vi "CAN_Simple_Demo.vi"() -> ()   [LabVIEW 2014]
uses:
  <vilib>/Utility/miscctls.llb/LVPointTypeDef.ctl
  Utilities/Global/DLL_Path.vi
  Utilities/Typedef/Hardware_Subtype.ctl
  TSMaster_API/CAN_CANFD_Function/Typedef/TSCAN_CAN_Configuration.ctl
  TSMaster_API/All_Control/Typedef/Hardware Type.ctl
panel:
  in  "Hardware Subtype":T1=enum."TC1016"
  in  "DLL_Path":path=path "D:/Program Files (x86)/TOSUN/TSMaster/bin/TSMaster.dll"
  out "ACANMsgBuffer":T2(array[cluster])
  out "Initialize array1":T2(array[cluster])
  out "Message&ID":string[](array[string])
  in  "Send":bool
  out "Initialize array":string[](array[string])
  out "ALLName":string[](array[string])
  out "SignalName":string[][](array[string])
  out "Message":string[](array[string])
  in  "tab control":enum32{"CANUI", "DBCUI"}(tab)
  in  "Data":T3 {"Data7" format="%x"; "Data6" format="%x"; "Data5" format="%x"; "Data4" format="%x"; "Data3" format="%x"; "Data2" format="%x"; "Data1" format="%x"; "Data0" format="%.0x"}
  in  "Length":u8
  in  "Frame type":u8(ring) items=["Data Frame", "Remote Frame"]
  in  "Frame format":u8(ring) items=["Standard Frame", "Extended Frame"]
  in  "ID 2":i32 format="%x"
  in  "Channel select":u8(ring) items=["CHN1", "CHN2", "CHN3", "CHN4", "CHN5", "CHN6", "CHN7", "CHN8", "CHN9", "CHN10", "CHN11", "CHN12", "CHN13", "CHN14", "CHN15", "CHN16", "CHN17", "CHN18", "CHN19", "CHN20", "CHN21", "CHN22", "CHN23", "CHN24", "CHN25", "CHN26", "CHN27", "CHN28", "CHN29", "CHN30", "CHN31", "CHN32"]
  in  "Data":i32(listbox)=-1
  in  "READ":i32(listbox)
  in  "Tree control":string(tree)
  in  "DBC Path":path
  in  "DBC loading channel":i32(ring) items=["CHN1", "CHN2", "CHN3", "CHN4", "CHN5", "CHN6", "CHN7", "CHN8", "CHN9", "CHN10", "CHN11", "CHN12", "CHN13", "CHN14", "CHN15", "CHN16", "CHN17", "CHN18", "CHN19", "CHN20", "CHN21", "CHN22", "CHN23", "CHN24", "CHN25", "CHN26", "CHN27", "CHN28", "CHN29", "CHN30", "CHN31", "CHN32"]
  in  "WRITE":string[][](table)
  out "ID":i32[](array[numeric]) format="%x"
  out "Connect":bool
  in  "Baud rate setting":dbl=500.0 format="%#_g k"
  in  "Application logic channel":i32(ring) items=["CHN1", "CHN2", "CHN3", "CHN4", "CHN5", "CHN6", "CHN7", "CHN8", "CHN9", "CHN10", "CHN11", "CHN12", "CHN13", "CHN14", "CHN15", "CHN16", "CHN17", "CHN18", "CHN19", "CHN20", "CHN21", "CHN22", "CHN23", "CHN24", "CHN25", "CHN26", "CHN27", "CHN28", "CHN29", "CHN30", "CHN31", "CHN32"]
  in  "Physical channel":i32(ring) items=["CHN1", "CHN2", "CHN3", "CHN4", "CHN5", "CHN6", "CHN7", "CHN8", "CHN9", "CHN10", "CHN11", "CHN12", "CHN13", "CHN14", "CHN15", "CHN16", "CHN17", "CHN18", "CHN19", "CHN20", "CHN21", "CHN22", "CHN23", "CHN24", "CHN25", "CHN26", "CHN27", "CHN28", "CHN29", "CHN30", "CHN31", "CHN32"]
  in  "Terminator":u16(ring)=1 items=["Disable", "Enable"]
  in  "Mode":u16(ring) items=["Normal", "ListenOnly"]
  in  "Number of channels used":u16(ring)=1 items=["1 Channel"=1, "2 Channels"=2, "3 Channels"=3, "4 Channels"=4, "5 Channels"=5]
  in  "Read message type":u16(ring)=1 items=["Only read received messages", "Receive&send messages"]
  in  "Hardware on/off":bool
  in  "Exit":bool
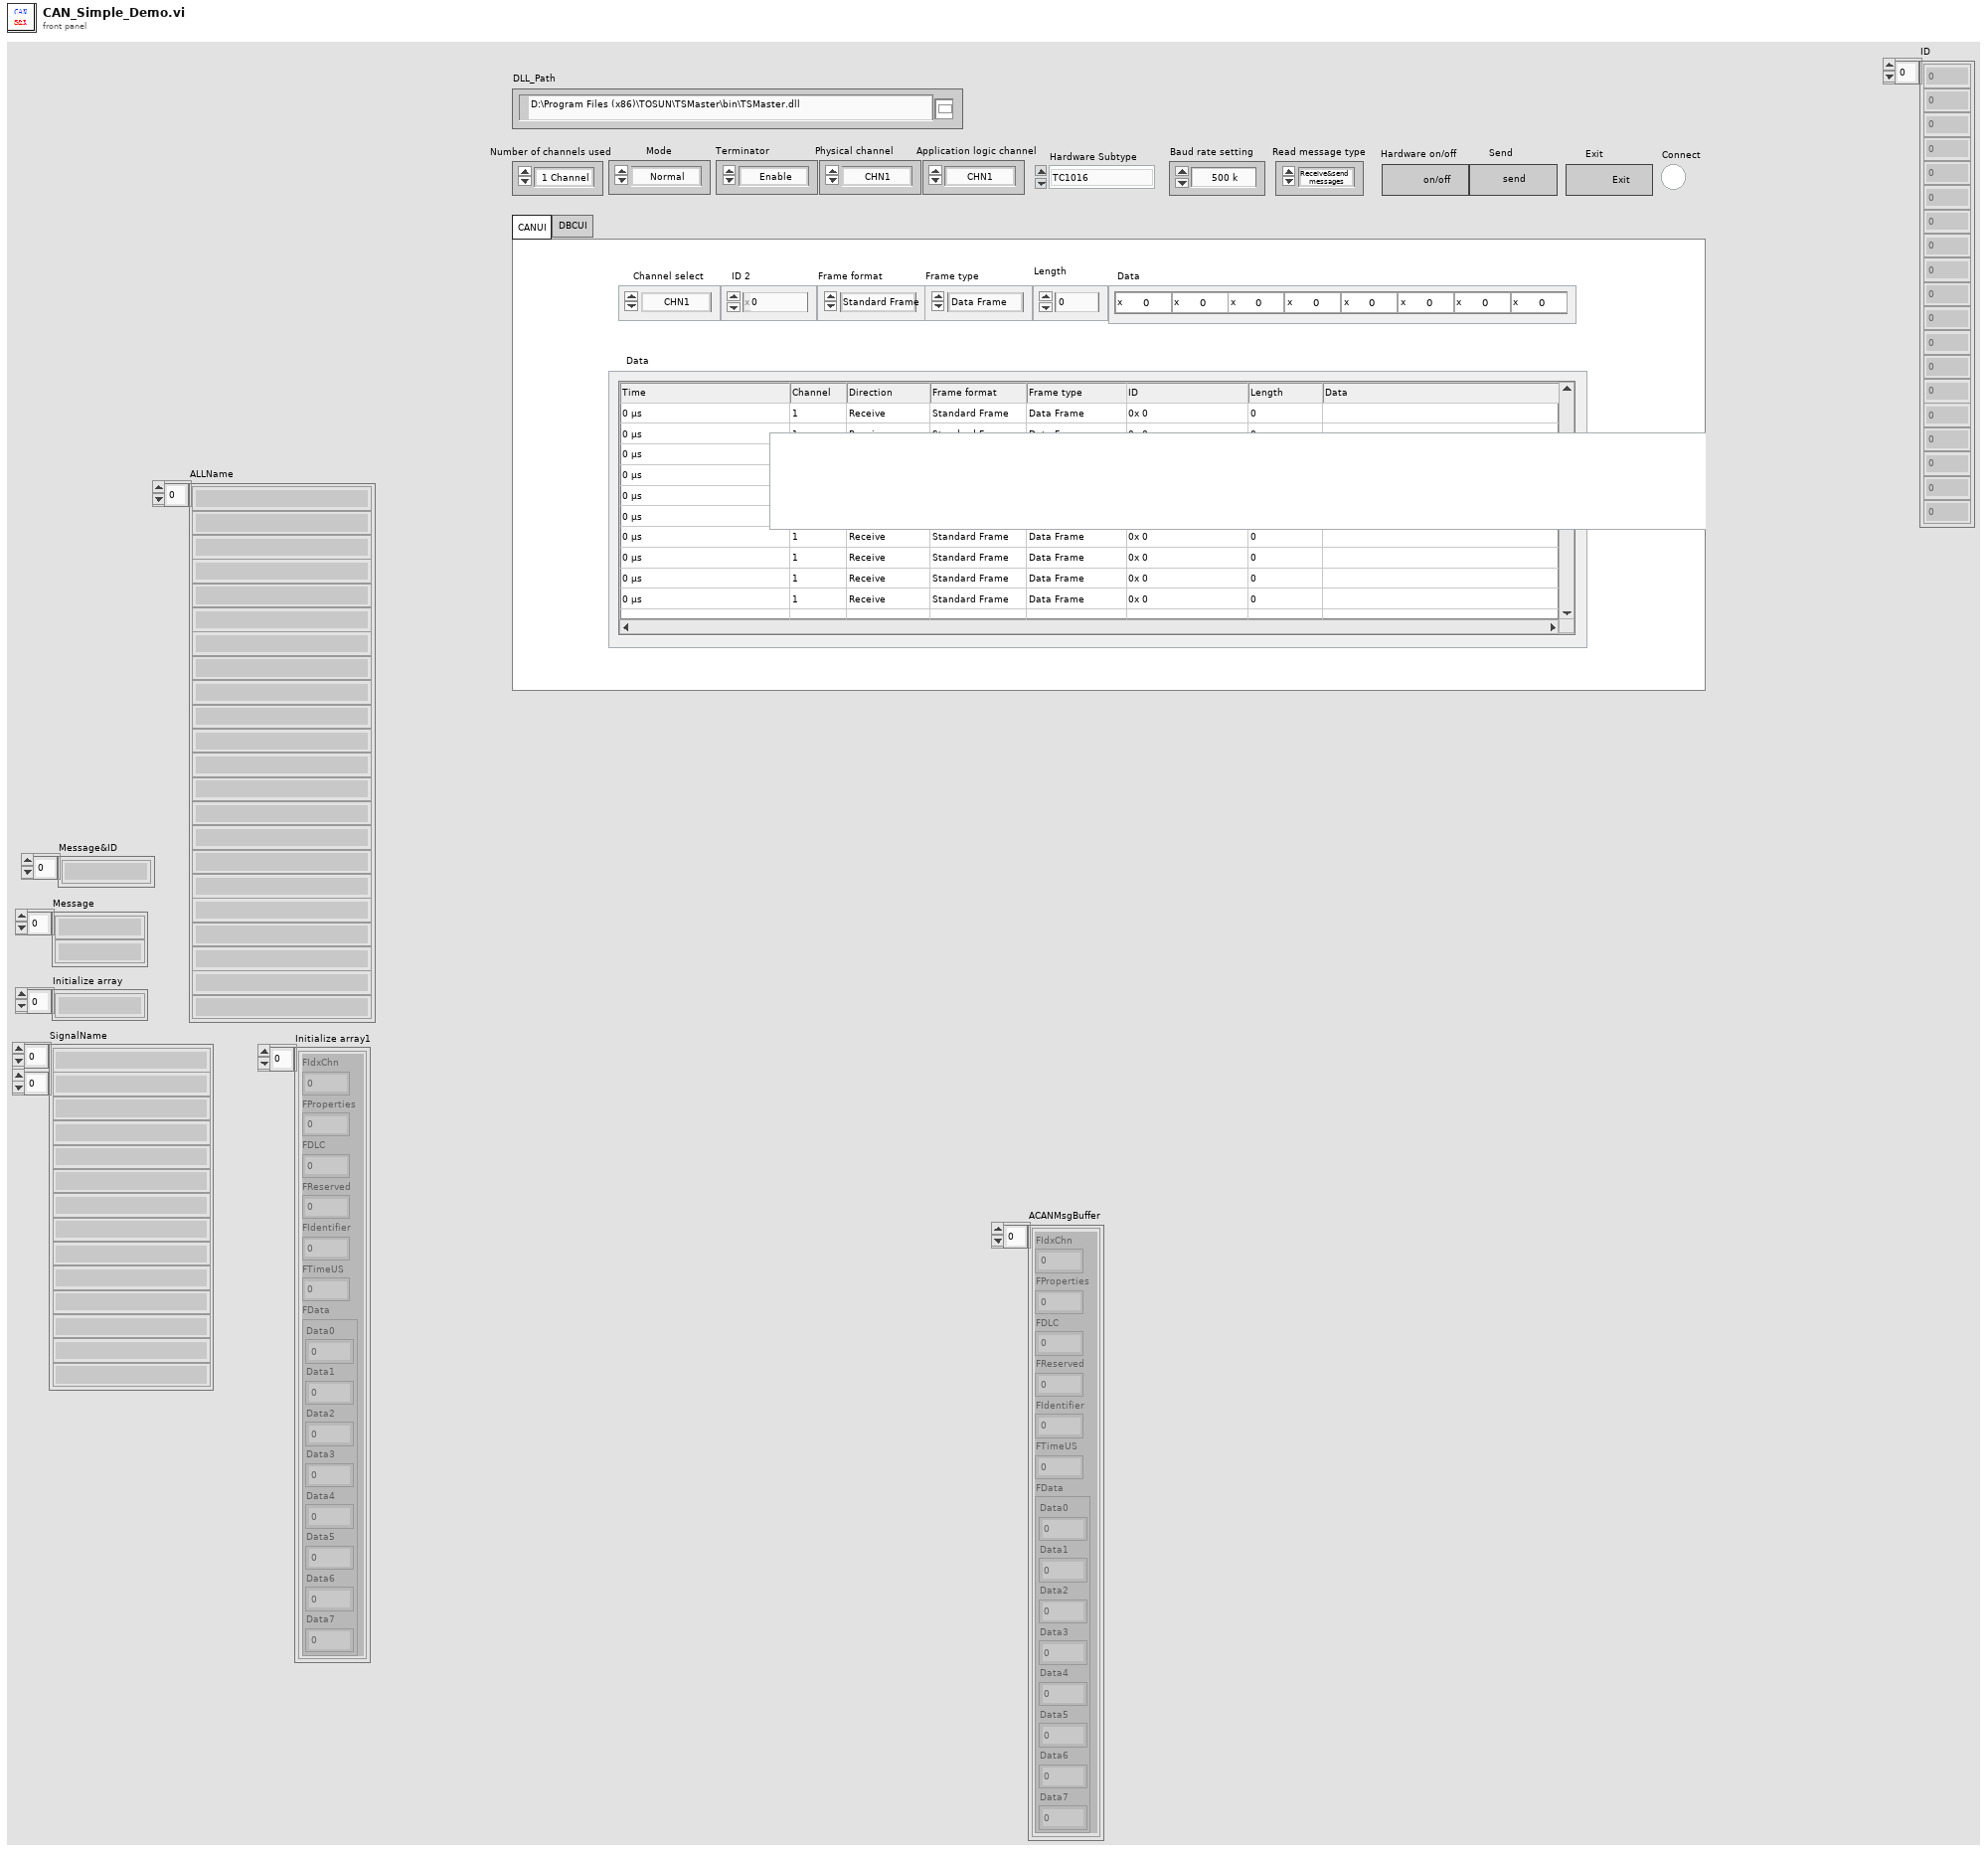
[diagram p1: front panel]
types:
  T1 = typedef "Hardware_Subtype.ctl" = enum16{"TS_UNKNOWN_DEVICE", "TSCAN_PRO", "TSCAN_Lite1", "TC1001", "TL1001", "TC1011", "TM5011", "TC1002", "TC1014", "TSCANFD2517", "TC1026", "TC1016", "TC1012", "TC1013", "TLog1002", "TC1034", "TC1018", "GW2116", "TC2115", "MP1013", "TC1113", "TC1114", "TP1013", "TC1017", "TP1018", "TF10XX", "TL1004_FD_4_LIN_2", "TE1051", "TP1051", "TP1034", "TTS9015", "TP1026", "TTS1026", "TTS1034", "TTS1018", "TL1011", "TTS1015_LiAuto", "TTS1013_LiAuto", "TTS1016Pro", "TC1054Pro", "TC1054", "TLog1038", "TO1013", "TC1034Pro", "TC1018Pro", "TC1038Pro", "TS_DEV_END"}
  T2 = cluster{"FIdxChn":u8, "FProperties":u8, "FDLC":u8, "FReserved":u8, "FIdentifier":i32, "FTimeUS":u64, "FData":cluster{"Data0":u8, "Data1":u8, "Data2":u8, "Data3":u8, "Data4":u8, "Data5":u8, "Data6":u8, "Data7":u8}}[]
  T3 = cluster{"Data0":u8, "Data1":u8, "Data2":u8, "Data3":u8, "Data4":u8, "Data5":u8, "Data6":u8, "Data7":u8}
  T4 = typedef "LVPointTypeDef.ctl" = cluster{"Horizontal":i16, "Vertical":i16}
  T5 = cluster{"FIdxChn":u8, "FProperties":u8, "FDLC":u8, "FReserved":u8, "FIdentifier":i32, "FTimeUS":u64, "FData":cluster{"Data0":u8, "Data1":u8, "Data2":u8, "Data3":u8, "Data4":u8, "Data5":u8, "Data6":u8, "Data7":u8}}
  T6 = typedef "TSCAN_CAN_Configuration.ctl" = cluster{"HardwareType":T7, "Hardware Subtype":T1, "ABaudrateKbps":sgl, "AListenOnly":enum16{"Normal", "ListenOnly"}, "Int120Ohm":enum16{"Disable", "Enable"}, "EnableChannel":enum16{"Disable", "Enable"}, "AHwChannel":i32, "AAppChannel":i32, "AldHW":i32}
  T7 = typedef "Hardware Type.ctl" = i32
  T8 = typedef "LVPoint32TypeDef.ctl" = cluster{"Horizontal":i32, "Vertical":i32}
  T9 = cluster{"Channel select":u8, "ID":i32, "Frame format":u8, "Frame type":u8, "Length":u8, "Data":cluster{"Data0":u8, "Data1":u8, "Data2":u8, "Data3":u8, "Data4":u8, "Data5":u8, "Data6":u8, "Data7":u8}}
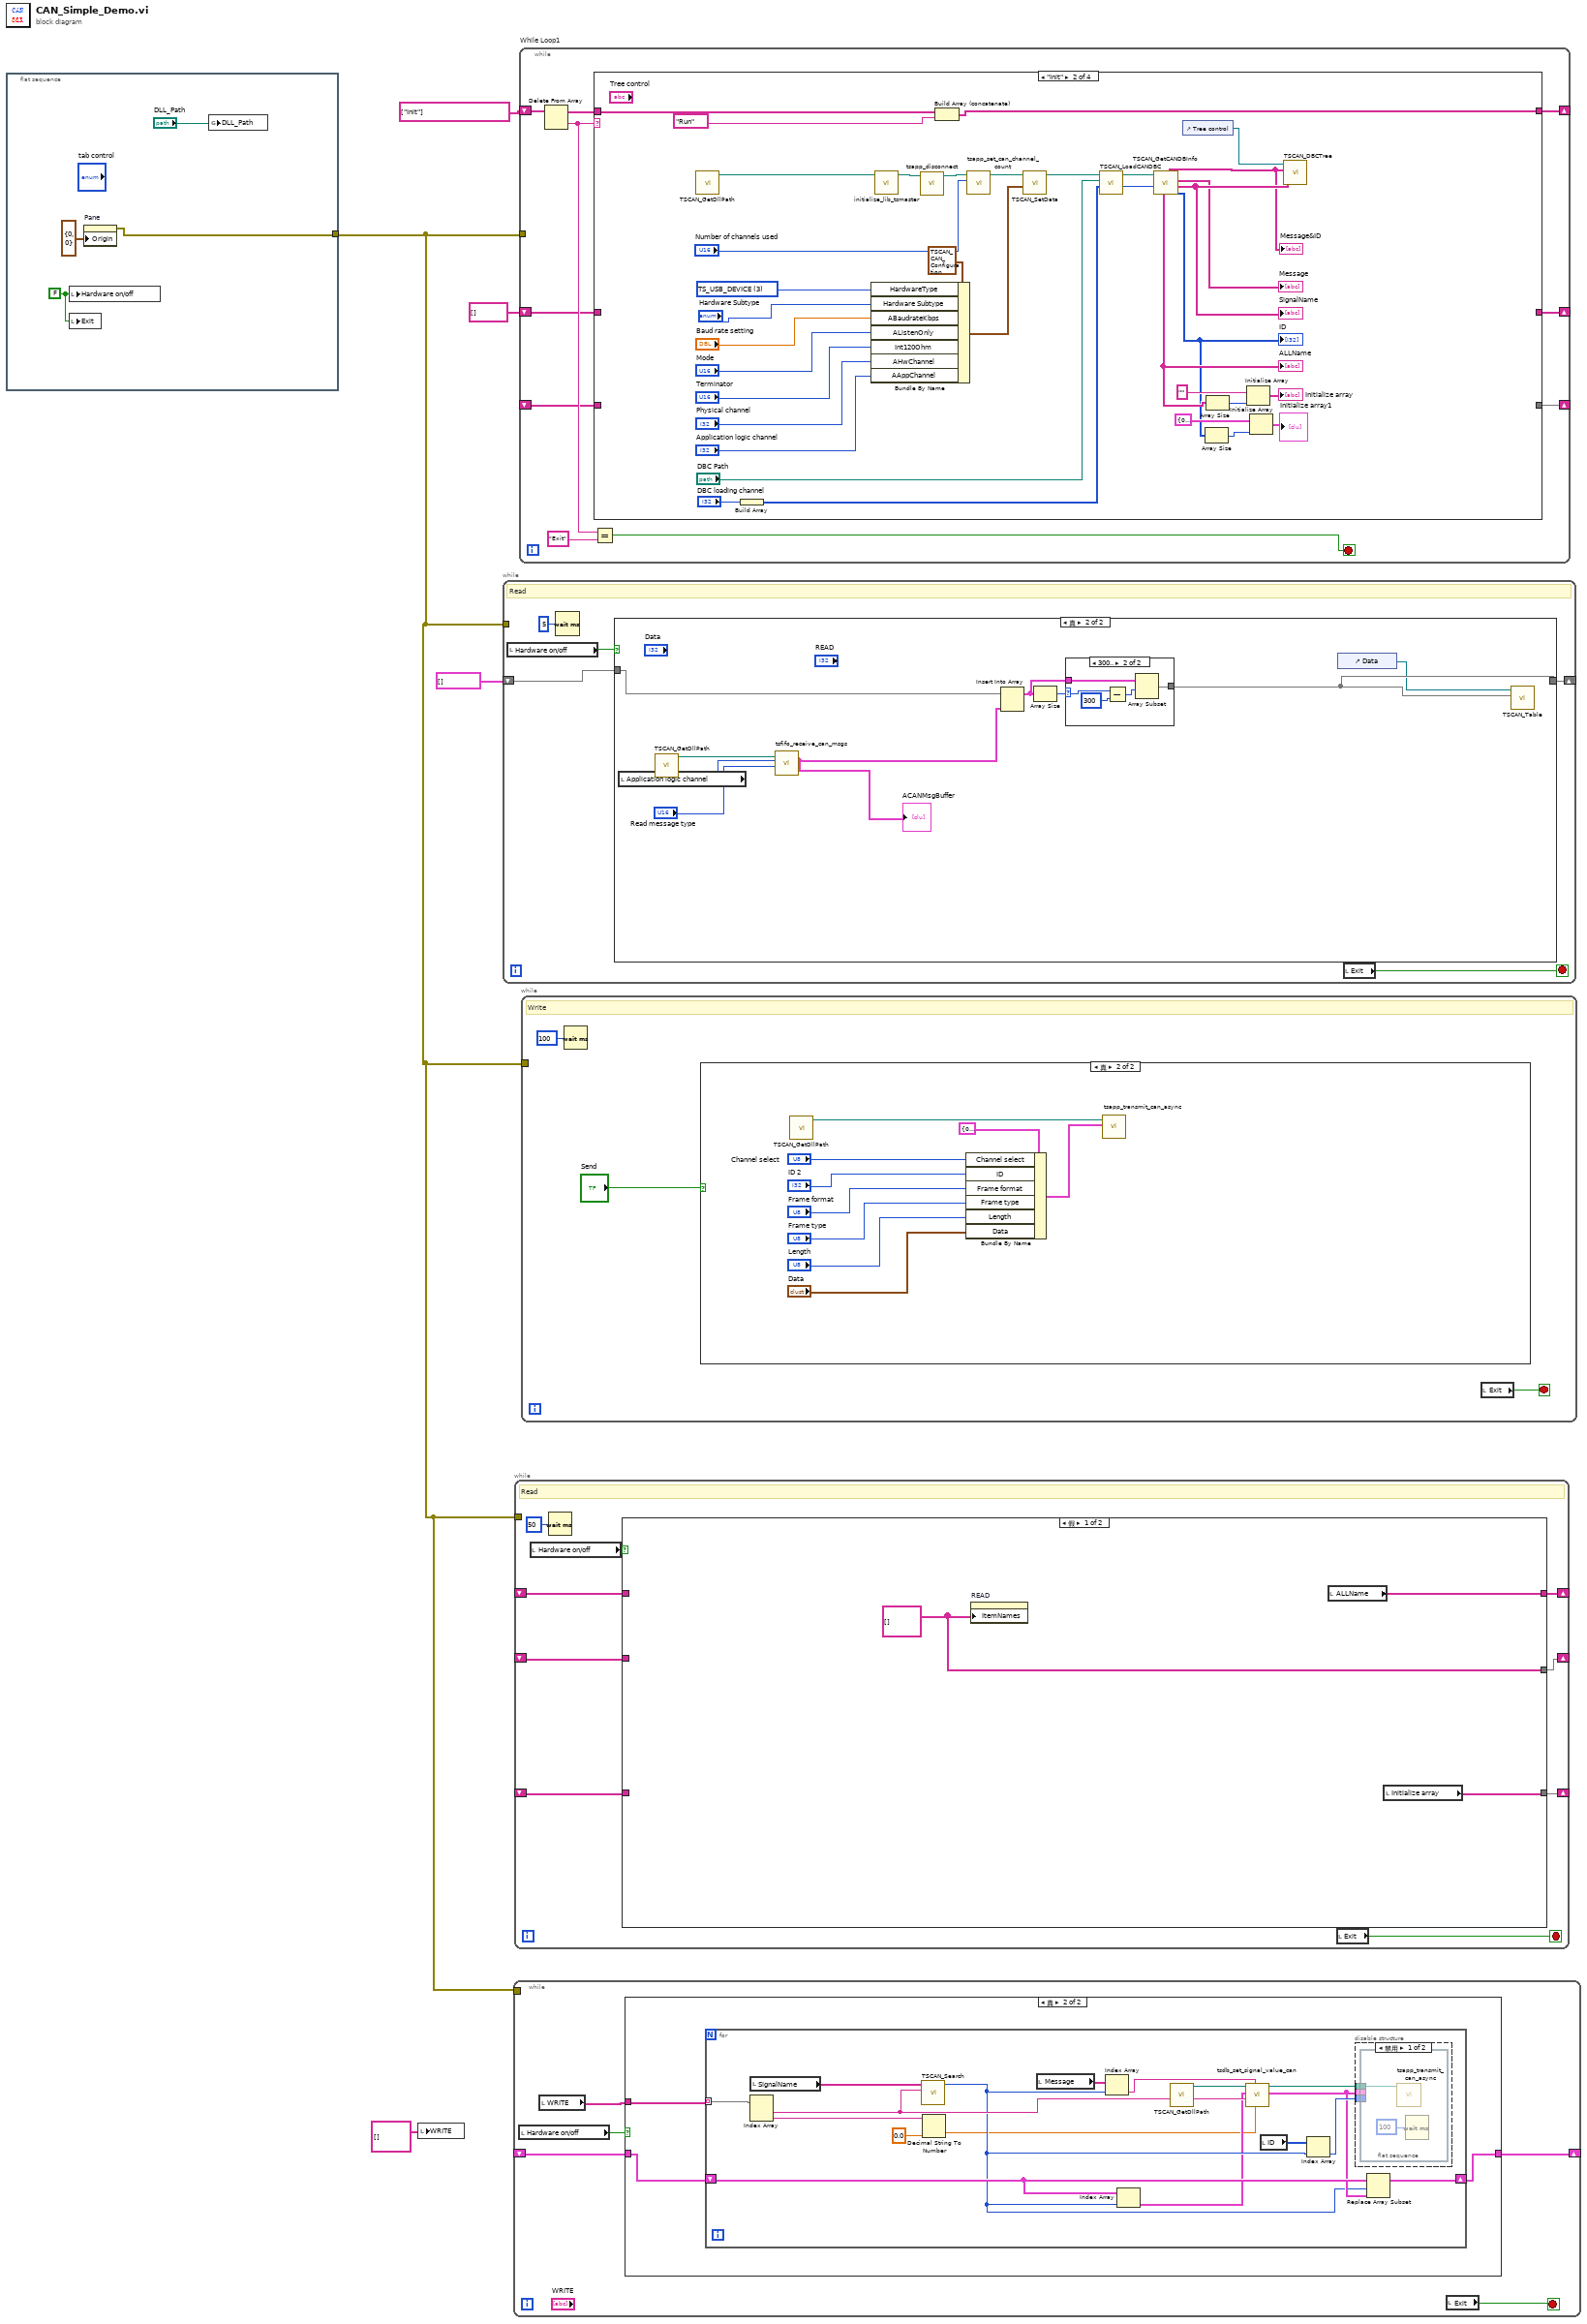
[diagram p0: block diagram]
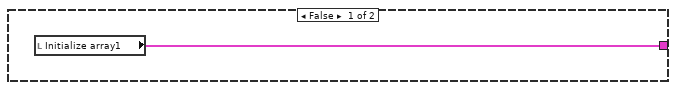
[diagram p2: hidden frame]
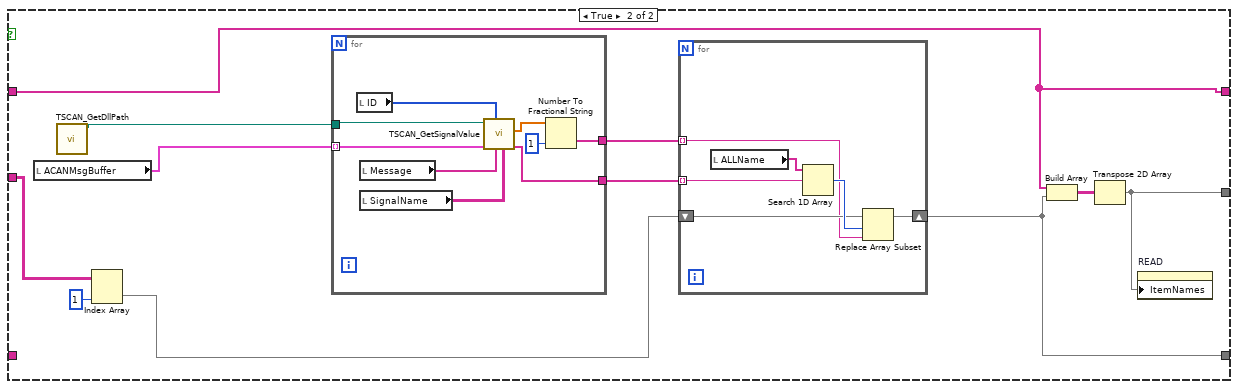
[diagram p4: hidden frame]
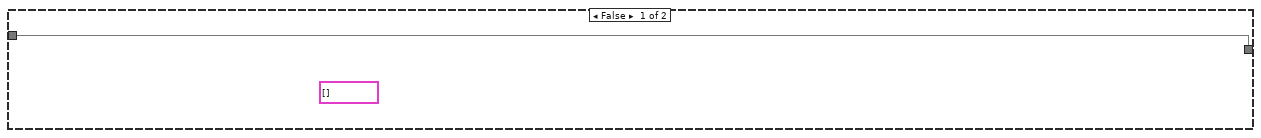
[diagram p6: hidden frame]
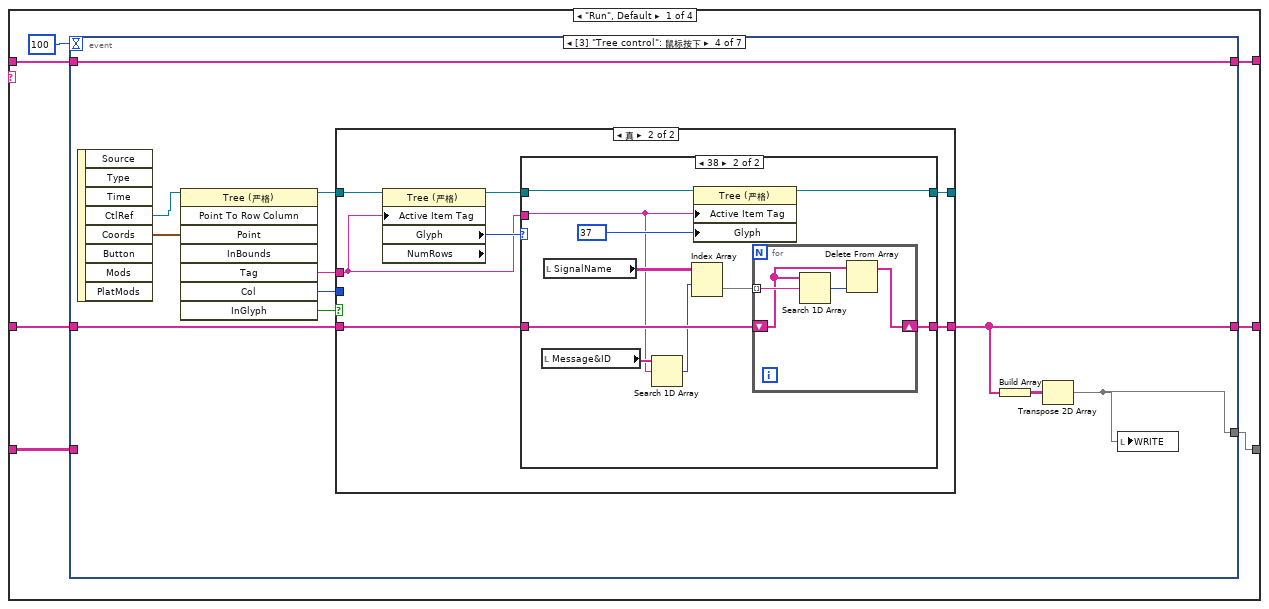
[diagram p8: hidden frame]
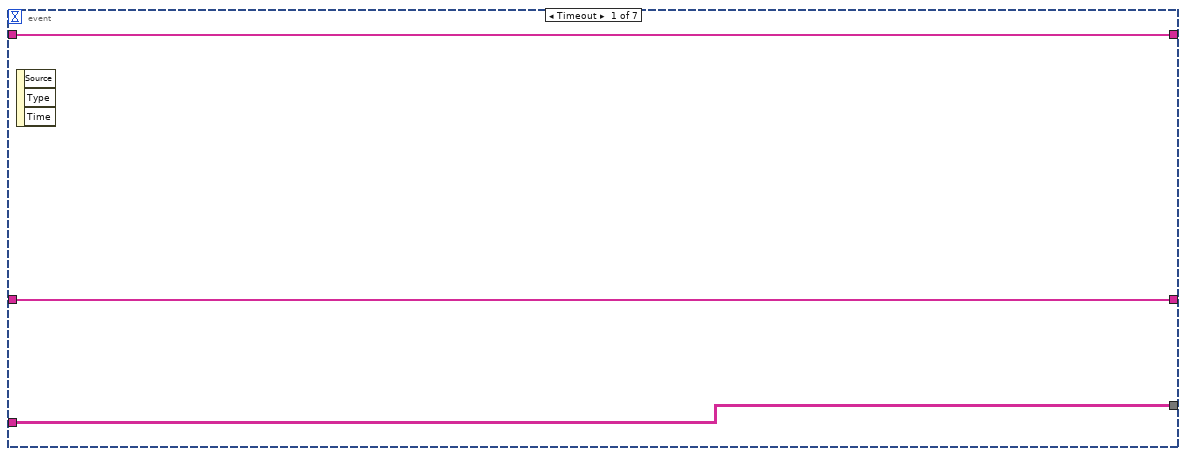
[diagram p9: hidden frame]
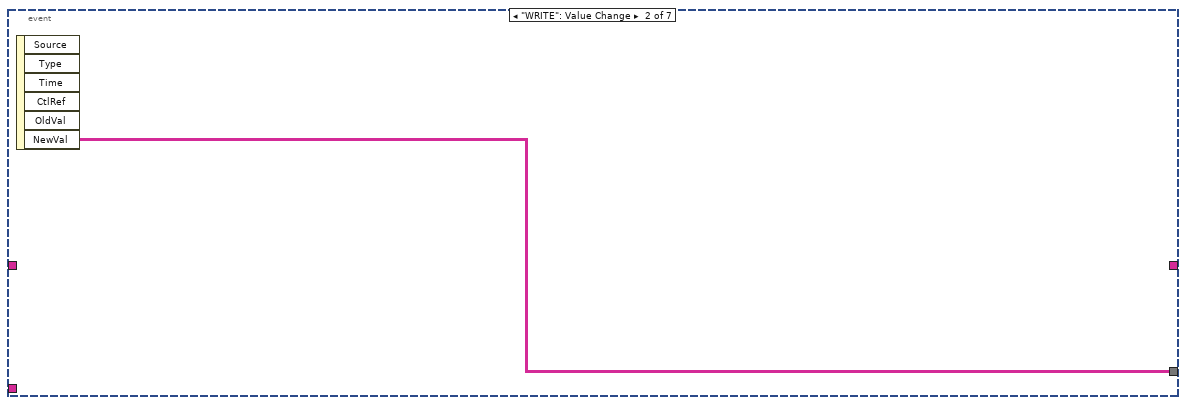
[diagram p10: hidden frame]
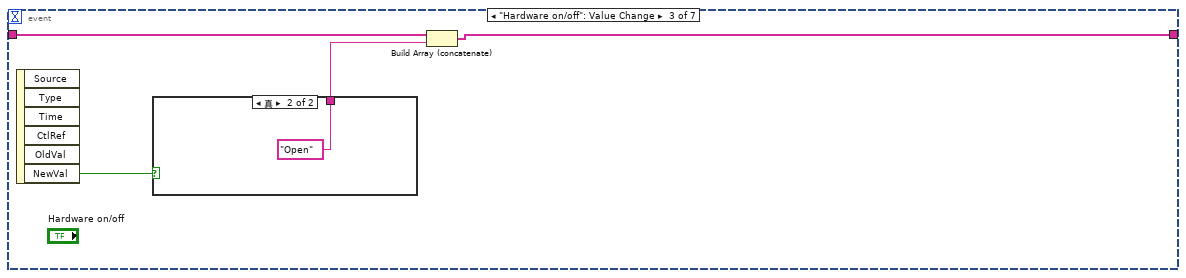
[diagram p11: hidden frame]
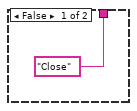
[diagram p12: hidden frame]
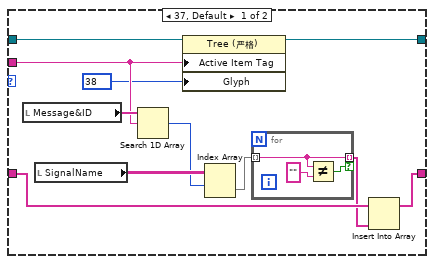
[diagram p14: hidden frame]
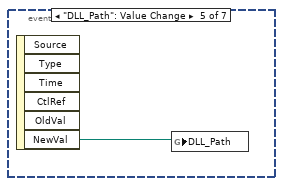
[diagram p15: hidden frame]
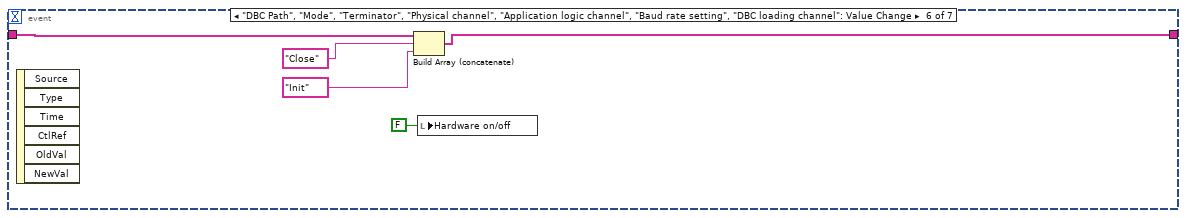
[diagram p16: hidden frame]
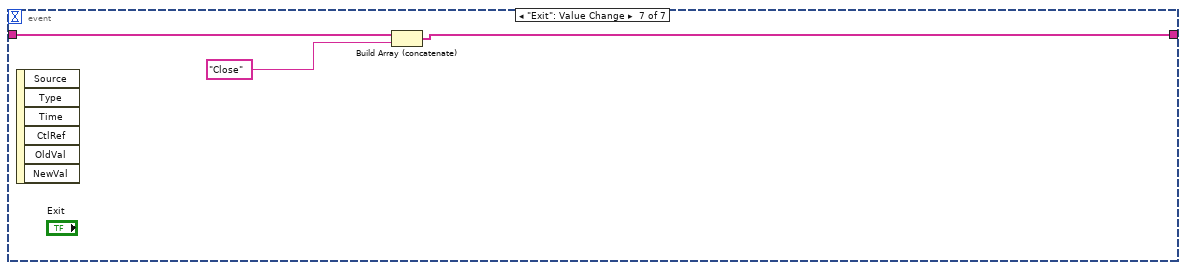
[diagram p17: hidden frame]
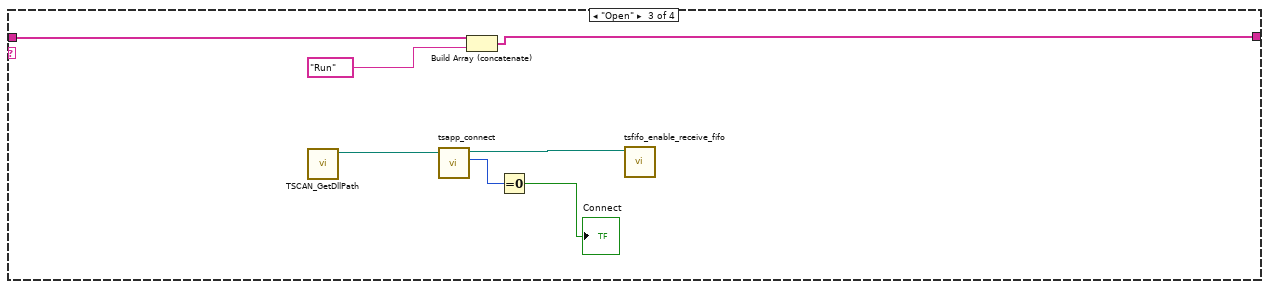
[diagram p18: hidden frame]
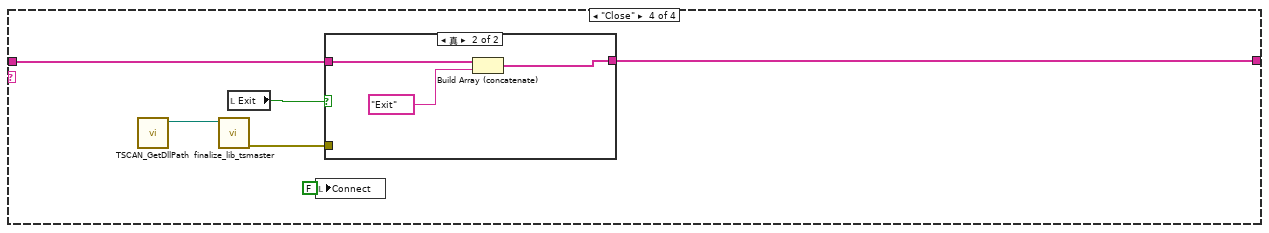
[diagram p19: hidden frame]
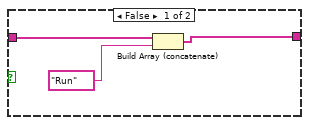
[diagram p20: hidden frame]
diagram:
  n1 = flat-sequence {
    tunnel: [w7] -> w1
    frame #0 {
      w9 = FALSE ("硬件启闭")
      n2 = local write "Hardware on/off"(w9) -> ()
      n3 = local write "Exit"(w9) -> ()
      n4 = property on="Pane" class="Pane"("Origin"=T4 {"Horizontal"=0, "Vertical"=0}) -> (error out=w7:errorcluster)  [unwired: 2 in, 1 out]
      n5 = global write "DLL_Path.vi" "DLL_Path"("DLL_Path") -> ()
    }
  }
  n6 = local write "WRITE"(string[][] [] ("WRITE")) -> ()
  n7 = while {
    shift-right: [w10] -> _
    shift-left: T2 [] ("数组") -> [w11]
    tunnel: w1 -> [_]
    stop <- w14 stop-if-true
    # "Read"
    n8 = local read "Hardware on/off"() -> (w12:bool)
    n9 = Wait (ms)(milliseconds to wait=u32 5 ("等待时间（毫秒）")) -> ()  [unwired: 1 out]
    n10 = case shown="真" w12 {
      tunnel: [w15 w19] -> w10
      tunnel: w11 -> [w15 w22]
      frame False {
        (unwired) T2 [] ("数组")
      }
      frame True {
        n11 = local read "Application logic channel"() -> (w23:i32)
        n12 = call "TSCAN_GetDllPath.vi"() -> ("DllPath"=w24:path)  [unwired: 11 in]
        n13 = call "tsfifo_receive_can_msgs.vi"("Read message type"="Read message type", "AAPPChannel"=w23, "Path"=w24) -> ("ACANMsgBuffer"=w16:T2)  [unwired: 4 in, 3 out]
        "ACANMsgBuffer" <- w16
        n14 = Insert Into Array(array=w22, new element=w16) -> (w20:T2)  [unwired: 1 in]
        n15 = Array Size(array=w20) -> (size(s)=w21:i32)
        n16 = case shown="300.." w21 {
          selector: w21 -> [_ w30]
          tunnel: [w25 w28] -> w19
          tunnel: w20 -> [w25 w26]
          frame 0, Default {
          }
          frame 300.. {
            n17 = Subtract(x=w30, y=300) -> (x-y=w27:i32)
            n18 = Array Subset(array=w26, index=w27) -> (w28:T2)  [unwired: 1 in]
          }
        }
        n19 = control-ref of="Data"() -> (w17:refnum<vi>)
        n20 = call "TSCAN_Table.vi"("Buffer"=w19, "MCListbox reference handle"=w17) -> ()  [unwired: 10 in]
      }
    }
    n21 = local read "Exit"() -> (w14:bool)
  }
  n22 = while {
    shift-right: [w33] -> _
    shift-left: _ -> [w32]
    tunnel: w1 -> [_]
    stop <- w35 stop-if-true
    n23 = local read "Hardware on/off"() -> (w34:bool)
    n24 = local read "WRITE"() -> (w31:string[][])
    n25 = case shown="真" w34 {
      tunnel: [w36 w38] -> w33
      tunnel: w32 -> [_ w39]
      tunnel: w31 -> [_ w37]
      frame False {
        n26 = local read "Initialize array1"() -> (w36:T2)
      }
      frame True {
        n27 = for {
          tunnel: w37 -> [w55] mode=indexing
          shift-right: [w44] -> w38
          shift-left: w39 -> [w46]
          n28 = Index Array(array=w55) -> (element #1=w47:string, element #2=w53:string)  [unwired: 2 in]
          n29 = local read "SignalName"() -> (w48:string[][])
          n30 = call "TSCAN_Search.vi"("字符串"=w47, "数组"=w48) -> ("数值"=w43:i32)  [unwired: 9 in]
          n31 = Decimal String To Number(string=w53, default (0L)=0.0 ("默认(0 I32)")) -> (number=w41:dbl)  [unwired: 1 in, 1 out]
          n32 = local read "Message"() -> (w54:string[])
          n33 = Index Array(array=w54, index=w43) -> (element=w40:string)
          n34 = Index Array(array=w46, index=w43) -> (element=w42:T5)
          n35 = call "TSCAN_GetDllPath.vi"() -> ("DllPath"=w56:path)  [unwired: 11 in]
          n36 = call "tsdb_set_signal_value_can.vi"("SigValue"=w41, "Signal Str"=w40, "Message"=w47, "CAN ObJ"=w42, "path"=w56) -> ("CANObJ"=w45:T5, "path out"=w51:path)  [unwired: 3 in, 2 out]
          n37 = local read "ID"() -> (w50:i32[])
          n38 = Index Array(array=w50, index=w43) -> (element=w49:i32)
          n39 = disable-structure shown="禁用" {
            disable-tunnel: w51 -> [w59 _]
            disable-tunnel: w49 -> [w58 _]
            disable-tunnel: w45 -> [w57 _]
            frame Disabled {
              n40 = flat-sequence {
                tunnel: w59 -> [w61]
                tunnel: w58 -> [_]
                tunnel: w57 -> [_]
                frame #0 {
                  n41 = call "tsapp_transmit_can_async.vi"("Path input"=w61) -> ()  [unwired: 8 in, 3 out]
                  n42 = Wait (ms)(milliseconds to wait=u32 100 ("等待时间（毫秒）")) -> ()  [unwired: 1 out]
                }
              }
            }
            frame Enabled {
            }
          }
          n43 = Replace Array Subset(array=w46, new element=w45, index=w43) -> (w44:T2)
        }
      }
    }
    n44 = local read "Exit"() -> (w35:bool)
  }
  n45 = while {
    shift-right: [w67] -> _
    shift-left: _ -> [w66]
    shift-right: [w65] -> _
    shift-left: _ -> [w64]
    shift-right: [w63] -> _
    shift-left: _ -> [w62]
    tunnel: w1 -> [_]
    stop <- w70 stop-if-true
    # "Read"
    n46 = local read "Hardware on/off"() -> (w68:bool)
    n47 = Wait (ms)(milliseconds to wait=u32 50 ("等待时间（毫秒）")) -> ()  [unwired: 1 out]
    n48 = case shown="假" w68 {
      tunnel: [w73 w80] -> w67
      tunnel: w66 -> [_ w79]
      tunnel: [w72 w81] -> w65
      tunnel: w64 -> [_ _]
      tunnel: [w71 w76] -> w63
      tunnel: w62 -> [_ w76]
      frame False {
        w73 = string[][] [] ("项名")
        n49 = property on="READ" class="MCListbox (严格)"("ItemNames"=w73) -> ()  [unwired: 2 in, 2 out]
        n50 = local read "ALLName"() -> (w71:string[])
        n51 = local read "Initialize array"() -> (w72:string[])
      }
      frame True {
        n52 = local read "ACANMsgBuffer"() -> (w74:T2)
        n53 = call "TSCAN_GetDllPath.vi"() -> ("DllPath"=w75:path)  [unwired: 11 in]
        n54 = Index Array(array=w79, index (col)=1 ("禁用的索引 (列)")) -> (element=w77:string[])  [unwired: 1 in]
        n55 = for {
          tunnel: w75 -> [w99]
          tunnel: w74 -> [w98] mode=indexing
          tunnel: [w97] -> w83
          tunnel: [w91] -> w82
          n56 = local read "ID"() -> (w96:i32[])
          n57 = local read "Message"() -> (w95:string[])
          n58 = local read "SignalName"() -> (w94:string[][])
          n59 = call "TSCAN_GetSignalValue.vi"("ALLSignalName"=w94, "ALLMessage"=w95, "ALLID"=w96, "簇"=w98, "path"=w99) -> ("array"=w97:string[], "SigValue"=w93:dbl[])  [unwired: 2 in, 3 out]
          n60 = Number To Fractional String(number=w93, precision (6)=i16 1 ("精度(6)")) -> (F-format string=w91:string[])  [unwired: 2 in]
        }
        n61 = for {
          tunnel: w83 -> [w90] mode=indexing
          tunnel: w82 -> [w86] mode=indexing
          shift-right: [w85] -> w81
          shift-left: w77 -> [w87]
          n62 = local read "ALLName"() -> (w89:string[])
          n63 = Search 1D Array(1D array=w89, element=w90) -> (index of element=w88:i32)  [unwired: 1 in]
          n64 = Replace Array Subset(array=w87, new element=w86, index=w88) -> (w85:string[])
        }
        n65 = Build Array(w76, w81) -> (w84:string[][])
        n66 = Transpose 2D Array(2D array=w84) -> (transposed array=w80:string[][])
        n67 = property on="READ" class="MCListbox (严格)"("ItemNames"=w80) -> ()  [unwired: 2 in, 2 out]
      }
    }
    n68 = local read "Exit"() -> (w70:bool)
  }
  n69 = while "While Loop1" {
    shift-right: [w107] -> _
    shift-left: string[] ["Init"] -> [w109]
    shift-right: [w102] -> _
    shift-left: string[] [] -> [w103]
    shift-right: [w100] -> _
    shift-left: _ -> [w101]
    tunnel: w1 -> [_]
    stop <- w104 stop-if-true
    n70 = Delete From Array(array=w109) -> (deleted portion=w106:string, array with subset deleted=w108:string[])  [unwired: 2 in]
    n71 = Equal?(x=w106, y="Exit") -> (x = y?=w104:bool)
    n72 = case shown="\"Init\"" w106 {
      tunnel: w108 -> [w115 w217 w222 w229]
      tunnel: [w114 w216 w221 w230] -> w107
      tunnel: w103 -> [w113 _ _ _]
      tunnel: [w112 _ _ _] -> w102
      tunnel: w101 -> [w111 _ _ _]
      tunnel: [w110 _ _ _] -> w100
      frame "Run", Default {
        n73 = event shown="[3] \"Tree control\": 鼠标按下" {
          selector: _ -> [_ _ _ _ _ _ _]
          dyn-events: _ -> [_ _ _ _ _ _ _]
          timeout: 100 -> [_ _ _ _ _ _ _]
          tunnel: w115 -> [w119 _ w124 w134 _ w180 w182]
          tunnel: [w119 _ w123 w134 _ w178 w181] -> w114
          tunnel: w113 -> [w118 _ _ w133 _ _ _]
          tunnel: [w118 _ _ w130 _ _ _] -> w112
          tunnel: w111 -> [w117 _ _ _ _ _ _]
          tunnel: [w117 w120 _ w127 _ _ _] -> w110
          event Timeout {
            n74 = event-data() -> ()  [unwired: 1 in, 3 out]
          }
          event "WRITE": Value Change {
            n75 = event-data() -> ("NewVal"=w120:string[][])  [unwired: 1 in, 5 out]
          }
          event "Hardware on/off": Value Change {
            n76 = event-data() -> ("NewVal"=w122:bool)  [unwired: 1 in, 5 out]
            n77 = case shown="真" w122 {
              tunnel: ["Close" "Open"] -> w121
              frame False {
              }
              frame True {
              }
            }
            n78 = Build Array (concatenate)(w124, w121) -> (w123:string[])
          }
          event "Tree control": Mouse Down {
            n79 = event-data() -> ("CtlRef"=w128:refnum<vi>, "Coords"=w135:T8)  [unwired: 1 in, 6 out]
            n80 = invoke class="Tree (严格)" method="Point To Row Column"(reference=w128, "Point"=w135) -> (reference out=w136:refnum<vi>, "Tag"=w132:string, "Col"=w131:i32, "InGlyph"=w137:bool)  [unwired: 6 in, 4 out]
            n81 = case shown="真" w137 {
              tunnel: w132 -> [_ w143]
              tunnel: w136 -> [w139 w146]
              tunnel: [w139 w142] -> _
              tunnel: w133 -> [w138 w141]
              tunnel: [w138 w140] -> w130
              tunnel: w131 -> [_ _]
              frame False {
              }
              frame True {
                n82 = property class="Tree (严格)" props=["Active Item Tag", "Glyph", "NumRows"](reference=w146, "Active Item Tag"=w143) -> (reference out=w144:refnum<vi>, "Glyph"=w145:i32)  [unwired: 1 in, 2 out]
                n83 = case shown="38" w145 {
                  tunnel: w144 -> [w154 w169]
                  tunnel: w143 -> [w152 w162]
                  tunnel: [w157 w168] -> w142
                  tunnel: w141 -> [w150 w166]
                  tunnel: [w155 w164] -> w140
                  frame 37, Default {
                    n84 = local read "Message&ID"() -> (w153:string[])
                    n85 = local read "SignalName"() -> (w156:string[][])
                    n86 = Search 1D Array(1D array=w153, element=w152) -> (index of element=w151:i32)  [unwired: 1 in]
                    n87 = property class="Tree (严格)"(reference=w154, "Active Item Tag"=w152, "Glyph"=38) -> (reference out=w157:refnum<vi>)  [unwired: 1 in, 1 out]
                    n88 = Index Array(array=w156, index (row)=w151) -> (element=w149:string[])  [unwired: 1 in]
                    n89 = for {
                      tunnel: w149 -> [w159] mode=indexing
                      tunnel: [w159] -> w148 mode=indexing if=w160
                      n90 = Not Equal?(x=w159, y="") -> (x != y?=w160:bool)
                    }
                    n91 = Insert Into Array(array=w150, new element=w148) -> (w155:string[])  [unwired: 1 in]
                  }
                  frame 38 {
                    n92 = local read "Message&ID"() -> (w163:string[])
                    n93 = local read "SignalName"() -> (w167:string[][])
                    n94 = Search 1D Array(1D array=w163, element=w162) -> (index of element=w161:i32)  [unwired: 1 in]
                    n95 = Index Array(array=w167, index (row)=w161) -> (element=w165:string[])  [unwired: 1 in]
                    n96 = property class="Tree (严格)"(reference=w169, "Active Item Tag"=w162, "Glyph"=37) -> (reference out=w168:refnum<vi>)  [unwired: 1 in, 1 out]
                    n97 = for {
                      shift-right: [w171] -> w164
                      shift-left: w166 -> [w172]
                      tunnel: w165 -> [w174] mode=indexing
                      n98 = Search 1D Array(1D array=w172, element=w174) -> (index of element=w173:i32)  [unwired: 1 in]
                      n99 = Delete From Array(array=w172, index=w173) -> (array with subset deleted=w171:string[])  [unwired: 1 in, 1 out]
                    }
                  }
                }
              }
            }
            n100 = Build Array(w130) -> (w129:string[][])
            n101 = Transpose 2D Array(2D array=w129) -> (transposed array=w127:string[][])
            n102 = local write "WRITE"(w127) -> ()
          }
          event "DLL_Path": Value Change {
            n103 = event-data() -> ("NewVal"=w175:path)  [unwired: 1 in, 5 out]
            n104 = global write "DLL_Path.vi" "DLL_Path"(w175) -> ()
          }
          event "DBC Path", "Mode", "Terminator", "Physical channel", "Application logic channel", "Baud rate setting", "DBC loading channel": Value Change {
            n105 = event-data() -> ()  [unwired: 1 in, 6 out]
            n106 = Build Array (concatenate)(w180, "Close", "Init") -> (w178:string[])
            n107 = local write "Hardware on/off"(FALSE ("硬件启闭")) -> ()
          }
          event "Exit": Value Change {
            n108 = event-data() -> ()  [unwired: 1 in, 6 out]
            n109 = Build Array (concatenate)(w182, "Close") -> (w181:string[])
          }
        }
      }
      frame "Init" {
        w192 = 3 items=["BUS_UNKNOWN_TYPE", "TS_TCP_DEVICE", "XL_USB_DEVICE", "TS_USB_DEVICE", "PEAK_USB_DEVICE", "KVASER_USB_DEVICE", "ZLG_USB_DEVICE", "ICS_USB_DEVICE", "TS_TC1005_DEVICE"] ("硬件类型")
        n110 = call "TSCAN_GetDllPath.vi"() -> ("DllPath"=w194:path)  [unwired: 11 in]
        n111 = Build Array("DBC loading channel") -> (w212:i32[])
        n112 = Bundle By Name(cluster=T6 {"HardwareType"=8, "Hardware Subtype"=enum."TC1016", "ABaudrateKbps"=250.0, "AListenOnly"=enum."Normal", "Int120Ohm"=enum."Enable", "EnableChannel"=enum."Enable", "AHwChannel"=0, "AAppChannel"=0, "AldHW"=0} ("CAN configuration"), "HardwareType"=w192, "Hardware Subtype"="Hardware Subtype", "ABaudrateKbps"="Baud rate setting", "AListenOnly"="Mode", "Int120Ohm"="Terminator", "AHwChannel"="Physical channel", "AAppChannel"="Application logic channel") -> (w185:T6)
        n113 = call "initialize_lib_tsmaster.vi"("Path input"=w194) -> ("Path output"=w195:path)  [unwired: 9 in, 1 out]
        n114 = call "tsapp_disconnect.vi"("Path"=w195) -> ("Path output"=w196:path)  [unwired: 8 in, 2 out]
        n115 = Build Array (concatenate)(w217, "Run") -> (w216:string[])
        n116 = call "tsapp_set_can_channel_count.vi"("Aount"="Number of channels used", "Path"=w196) -> ("Path output"=w197:path)  [unwired: 7 in, 2 out]
        n117 = call "TSCAN_SetData.vi"("CAN configuration"=w185, "Path"=w197) -> ("Path output"=w215:path)  [unwired: 6 in, 3 out]
        n118 = call "TSCAN_LoadCANDBC.vi"("ABindChannels"=w212, "ADBCAbsolutePath"="DBC Path", "Path"=w215) -> ("AIdOut"=w210:u32, "Path output"=w211:path)  [unwired: 5 in, 2 out]
        n119 = call "TSCAN_GetCANDBInfo.vi"("ADatabaseld"=w210, "Path"=w211) -> ("ID"=w199:i32[], "SignalName"=w208:string[][], "Message"=→"Message":string[], "Message&ID"=w207:string[], "ALLName"=w204:string[])  [unwired: 3 in, 1 out]
        "ID" <- w199
        "SignalName" <- w208
        "ALLName" <- w204
        "Message&ID" <- w207
        n120 = control-ref of="Tree control"() -> (w209:refnum<vi>)
        n121 = Array Size(array=w199) -> (size(s)=w200:i32)
        n122 = Array Size(array=w204) -> (size(s)=w205:i32)
        n123 = Initialize Array("", w205) -> (→"Initialize array":string[])
        n124 = Initialize Array(T5 {"FIdxChn"=0, "FProperties"=0, "FDLC"=0, "FReserved"=0, "FIdentifier"=0, "FTimeUS"=0, "FData"={"Data0"=0, "Data1"=0, "Data2"=0, "Data3"=0, "Data4"=0, "Data5"=0, "Data6"=0, "Data7"=0}} ("CANObJ"), w200) -> (→"Initialize array1":T2)
        n125 = call "TSCAN_DBCTree.vi"("child node"=w208, "Parent node"=w207, "control"=w209) -> ()  [unwired: 9 in]
      }
      frame "Open" {
        n126 = call "TSCAN_GetDllPath.vi"() -> ("DllPath"=w224:path)  [unwired: 11 in]
        n127 = call "tsapp_connect.vi"("Path"=w224) -> ("retuen"=w220:i32, "Path output"=w225:path)  [unwired: 8 in, 1 out]
        n128 = Build Array (concatenate)(w222, "Run") -> (w221:string[])
        n129 = Equal To 0?(x=w220) -> (x = 0?=→"Connect":bool)
        n130 = call "tsfifo_enable_receive_fifo.vi"("Path"=w225) -> ()  [unwired: 9 in, 2 out]
      }
      frame "Close" {
        n131 = call "TSCAN_GetDllPath.vi"() -> ("DllPath"=w228:path)  [unwired: 11 in]
        n132 = call "finalize_lib_tsmaster.vi"("Path"=w228) -> ("error out"=w227:errorcluster)  [unwired: 9 in, 1 out]
        n133 = local read "Exit"() -> (w231:bool)
        n134 = local write "Connect"(FALSE ("通讯")) -> ()
        n135 = case shown="真" w231 {
          tunnel: [w232 w236] -> w230
          tunnel: w229 -> [w233 w235]
          tunnel: w227 -> [_ _]
          frame False {
            n136 = Build Array (concatenate)(w233, "Run") -> (w232:string[])
          }
          frame True {
            n137 = Build Array (concatenate)(w235, "Exit") -> (w236:string[])
          }
        }
      }
    }
  }
  n138 = while {
    tunnel: w1 -> [_]
    stop <- w240 stop-if-true
    # "Write"
    n139 = Wait (ms)(milliseconds to wait=u32 100 ("等待时间（毫秒）")) -> ()  [unwired: 1 out]
    n140 = case shown="真" "Send" {
      frame False {
      }
      frame True {
        n141 = call "TSCAN_GetDllPath.vi"() -> ("DllPath"=w249:path)  [unwired: 11 in]
        n142 = Bundle By Name(cluster=T9 {"Channel select"=0, "ID"=274, "Frame format"=0, "Frame type"=0, "Length"=3, "Data"={"Data0"=11, "Data1"=0, "Data2"=0, "Data3"=0, "Data4"=0, "Data5"=0, "Data6"=0, "Data7"=0}} ("TCAN"), "Channel select"="Channel select", "ID"="ID 2", "Frame format"="Frame format", "Frame type"="Frame type", "Length"="Length", "Data"="Data") -> (w242:T9)
        n143 = call "tsapp_transmit_can_async.vi"("TCAN"=w242, "Path input"=w249) -> ()  [unwired: 7 in, 3 out]
      }
    }
    n144 = local read "Exit"() -> (w240:bool)
  }
